vi "Smart Subtraction.vi"(10 "y":dbl, 11 "x":dbl) -> (3 "x-y":dbl)   [LabVIEW 2018]
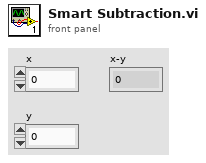
[diagram p1: front panel]
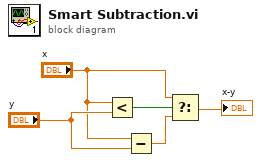
[diagram p0: block diagram]
diagram:
  n1 = Less?(x="x", y="y") -> (x < y?=w1:bool)
  n2 = Subtract(x="x", y="y") -> (x-y=w4:dbl)
  n3 = Select(t="x", s=w1, f=w4) -> (s? t:f=→"x-y":dbl)
